vi "Write Scale.vi"(5 "Scale":refnum<class "Scale.lvclass">, 9 "Knob in":refnum<class "Knob.lvclass">) -> (3 "Knob out":refnum<class "Knob.lvclass">)   [LabVIEW 2014, in "Knob.lvclass"]
uses:
  Knob.lvclass
  Scale/Scale.lvclass
  Knob.lvclass/Knob.ctl
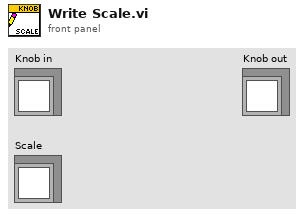
[diagram p1: front panel]
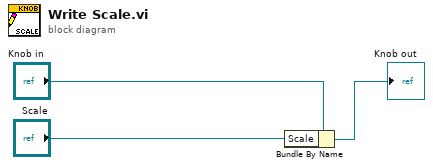
[diagram p0: block diagram]
diagram:
  n1 = Bundle By Name(cluster="Knob in", "Scale"="Scale") -> (→"Knob out":refnum<class "Knob.lvclass">)
